vi "Parameter Set Read Array.vi"(8 "error in":errorcluster, 11 "Cycler in":refnum<class "Cycler.lvclass">) -> (0 "error out":errorcluster, 1 "Changed or First Call?":bool, 2 "Parameter Set CTL":i32[](array[numeric]), 3 "Cycler out":refnum<class "Cycler.lvclass">)   [LabVIEW 2023, in "Cycler.lvclass"]
uses:
  Cycler.lvclass
  Cycler.lvclass/Cycler.ctl
  Low Level Capabilities/Parameter Set/Parameter Set.lvclass
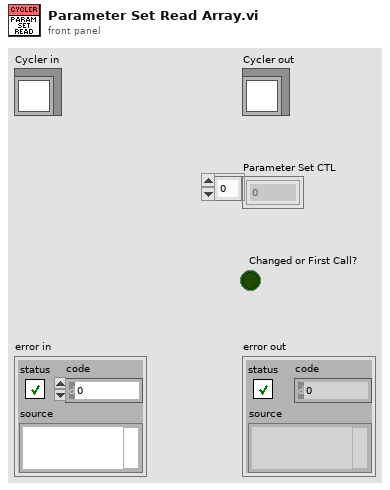
[diagram p1: front panel]
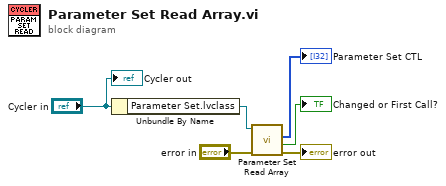
[diagram p0: block diagram]
diagram:
  n1 = Unbundle By Name("Cycler in") -> ("Parameter Set.lvclass"=w5:refnum<class "Parameter Set.lvclass">)
  n2 = call-dynamic "Parameter Set Read Array.vi"("error in (no error)"="error in", "Parameter Set in"=w5) -> ("error out"=→"error out":errorcluster, "Changed or First Call?"=→"Changed or First Call?":bool, "Parameter Set CTL"=→"Parameter Set CTL":i32[])  [unwired: 6 in, 1 out]
  "Cycler out" <- "Cycler in"
